vi "DestroyMessageQueues.vi"(8 "error in (no error)":errorcluster, 11 "queue in":T1[](array[typedef])) -> (0 "error out":errorcluster)   [LabVIEW 2020, in "MessageQueue.lvlib"]
doc: "Destroys (multiple) queue(s) created by CreateMessageQueue.vi"
uses:
  MessageQueue.lvlib
  QueueRef.ctl
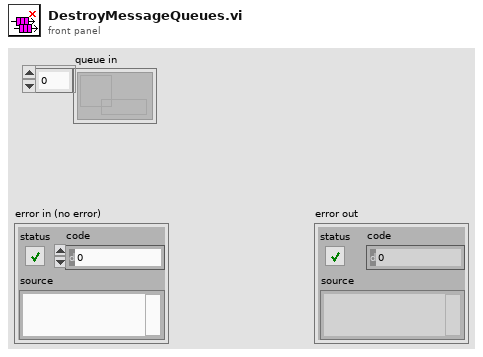
[diagram p1: front panel]
types:
  T1 = typedef "MessageQueue.lvlib/QueueRef.ctl" = refnum<queue>
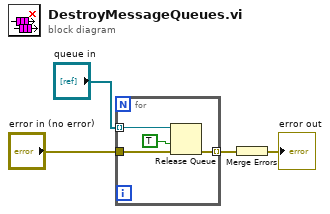
[diagram p0: block diagram]
diagram:
  n1 = for {
    tunnel: "queue in" -> [w8] mode=indexing
    tunnel: "error in (no error)" -> [w7]
    tunnel: [w6] -> w2 mode=indexing
    n2 = Release Queue(queue=w8, force destroy? (F)=TRUE, error in (no error)=w7) -> (error out=w6:errorcluster)  [unwired: 2 out]
  }
  n3 = Merge Errors(w2) -> (→"error out":errorcluster)
